vi "grey--constant.vi"() -> (1 "Gray":u32(colorbox))   [LabVIEW 2018, in "Resistor Band Colors.lvlib"]
uses:
  Resistor Band Colors.lvlib
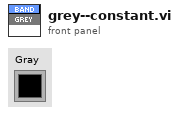
[diagram p1: front panel]
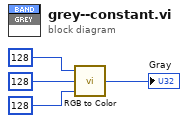
[diagram p0: block diagram]
diagram:
  n1 = call <vilib>:"RGB to Color.vi"("B"=u8 128, "G"=u8 128, "R"=u8 128) -> ("Color"=→"Gray":u32)
